vi "P26_Ilum_LDR.vi"() -> ()   [LabVIEW 2022 SP3]
panel:
  out "Boolean":bool
  in  "V de encendido":dbl
  out "Voltaje LDR":dbl
  in  "stop":bool
  # "P18a_An_In"
  # "Equipo C\nJairo Issac García López\nRodolfo Durón Hernandez\nRoberto Carlos Herrera Pérez\nSebastián Rodríguez Posada"
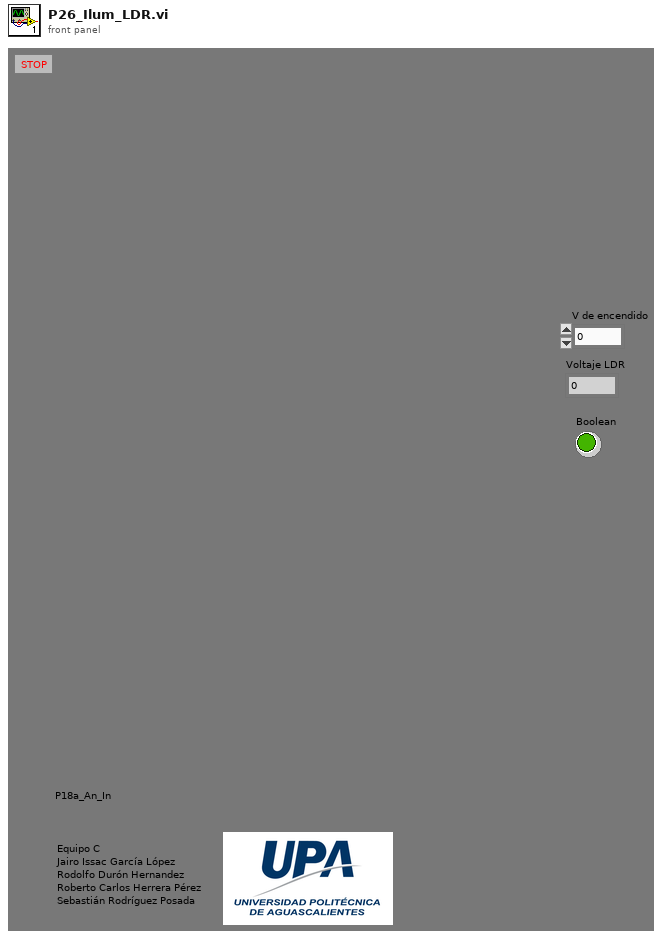
[diagram p1: front panel]
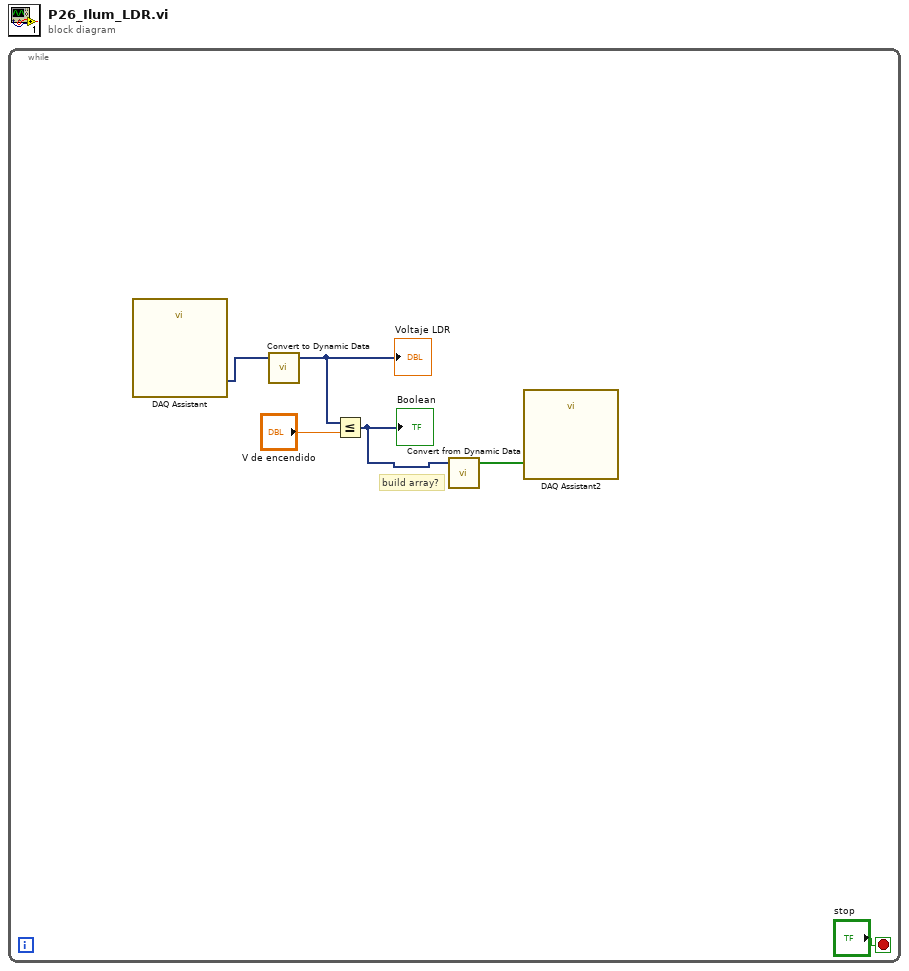
[diagram p0: block diagram]
diagram:
  n1 = while {
    stop <- "stop" stop-if-true
    # "build array?"
    n2 = call "DAQ Assistant"() -> ("data"=w4:dynamicdata)  [unwired: 17 in, 2 out]
    n3 = call "Convert to Dynamic Data"("Double"=w4) -> ("Dynamic Data Type"=w3:dynamicdata)  [unwired: 3 in]
    "Voltaje LDR" <- w3
    n4 = Less Or Equal?(x=w3, y="V de encendido") -> (x <= y?=w2:dynamicdata)
    "Boolean" <- w2
    n5 = call "Convert from Dynamic Data"("Dynamic Data Type"=w2) -> ("Array"=w1:bool[])  [unwired: 3 in]
    n6 = call "DAQ Assistant2"("data"=w1) -> ()  [unwired: 17 in, 2 out]
  }
